vi "S2C_BldQuickView.vi"(8 "Error In":errorcluster) -> (0 "Error Out":errorcluster)   [LabVIEW 2015]
doc: "Detects an error and calls the error case to process the error."
uses:
  Globals/S2C_Globals.vi
  Globals/S2C_GlobalMenus.vi
panel:
  in  "QV-Exit":bool
  out "Init":bool
  in  "Selection":enum16{"Command", "Step", "Both"}(ring)=enum."Both"
  out "Window":string
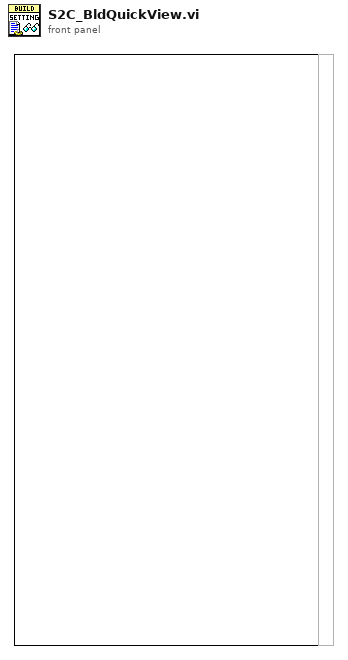
[diagram p1: front panel]
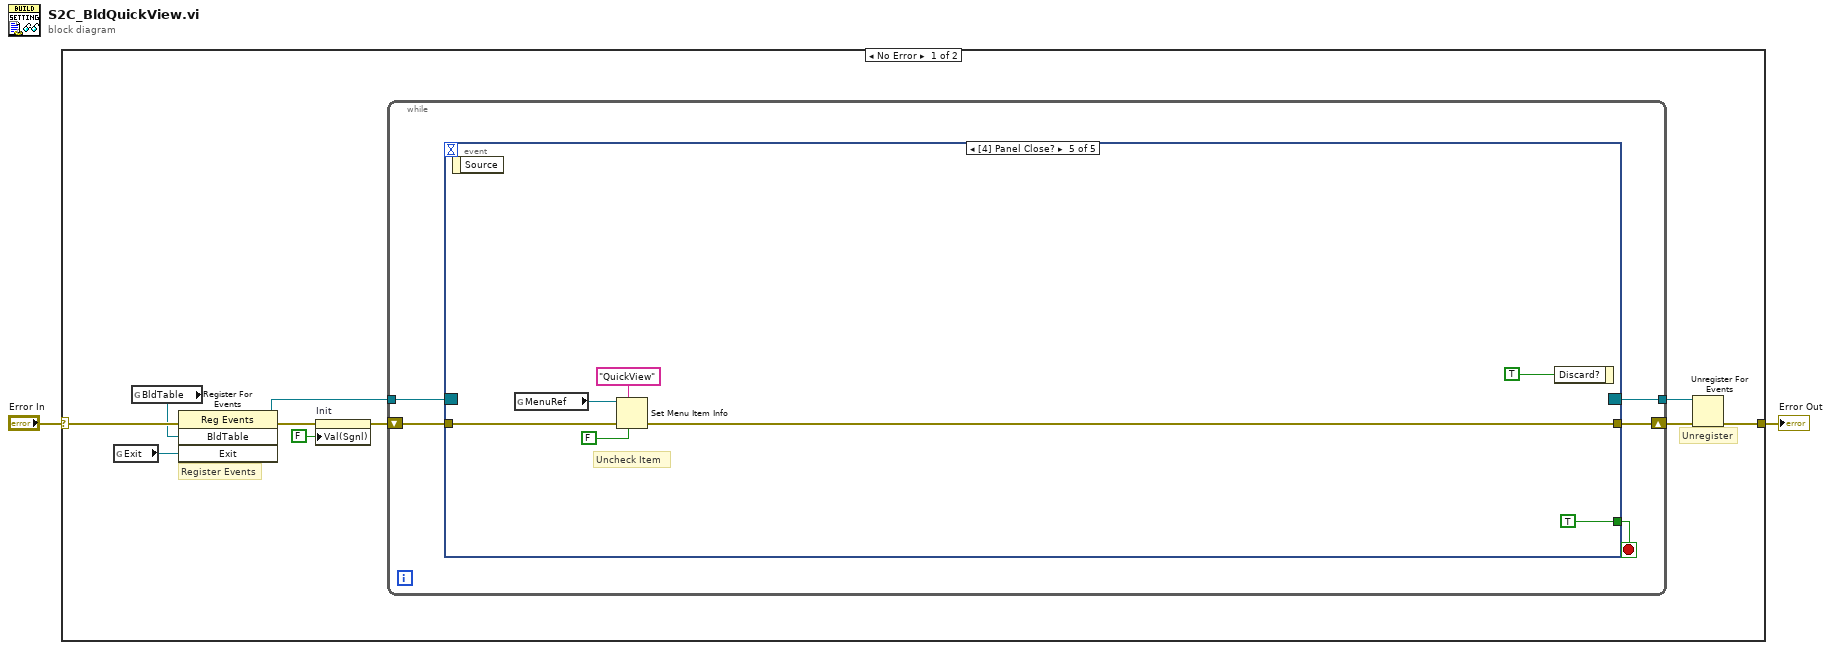
[diagram p0: block diagram]
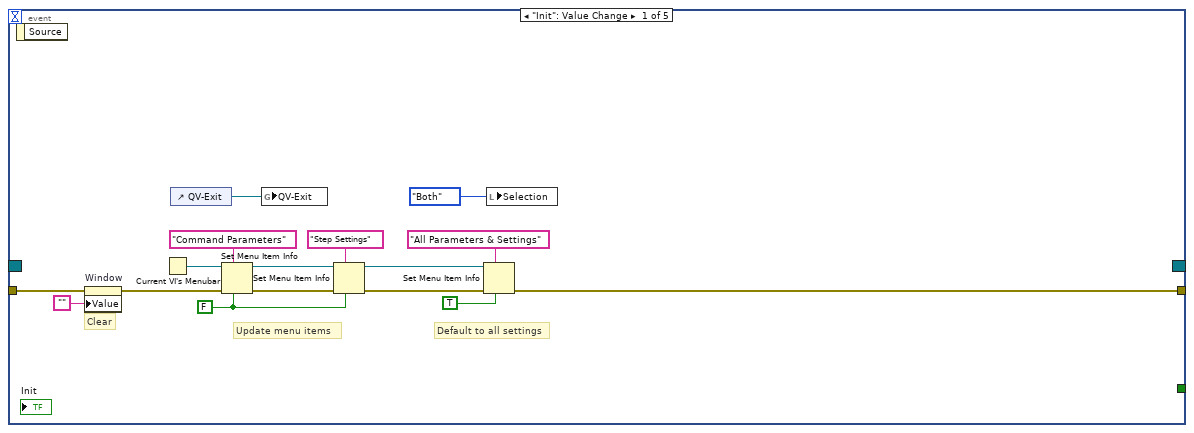
[diagram p2: hidden frame]
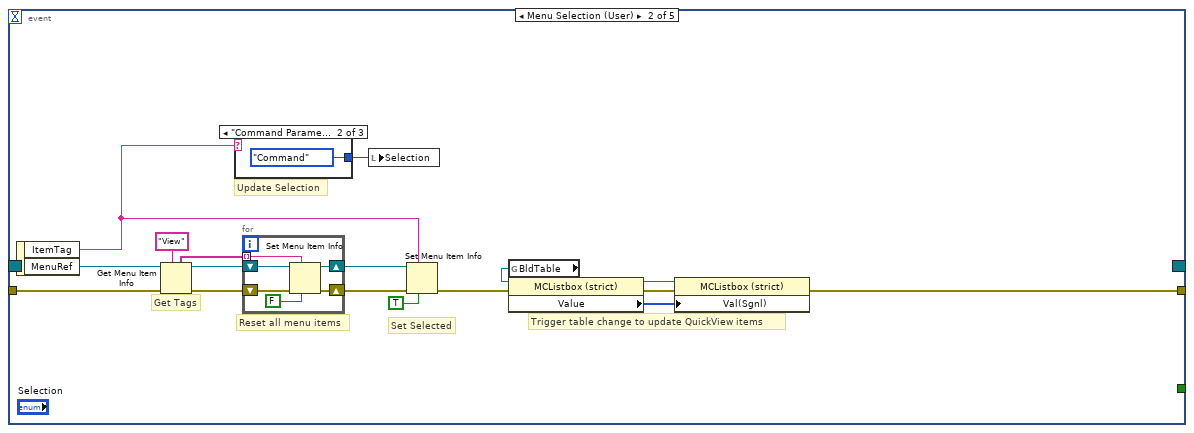
[diagram p3: hidden frame]
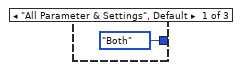
[diagram p4: hidden frame]
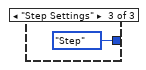
[diagram p5: hidden frame]
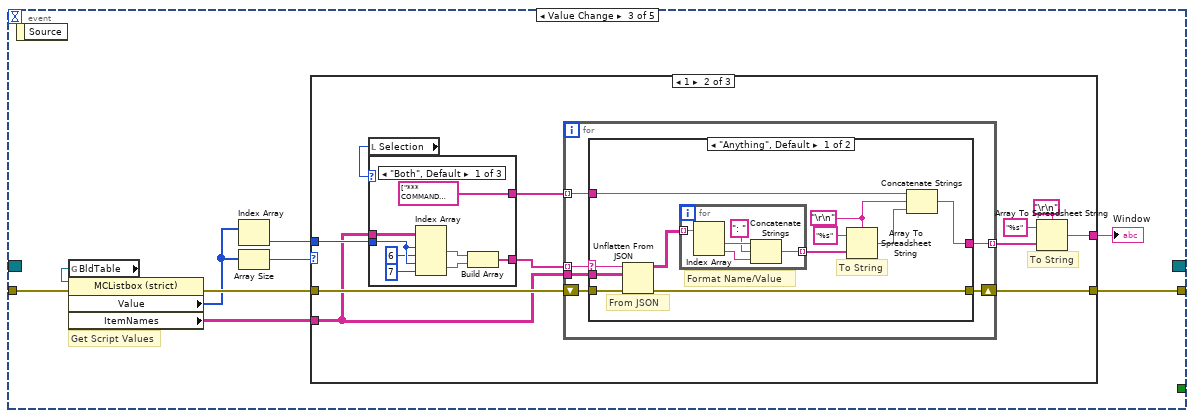
[diagram p6: hidden frame]
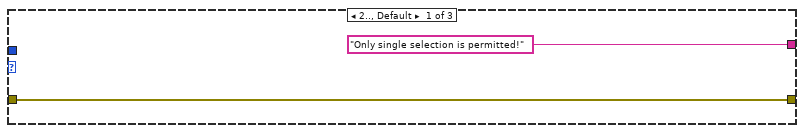
[diagram p7: hidden frame]
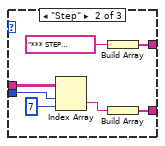
[diagram p8: hidden frame]
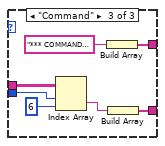
[diagram p9: hidden frame]
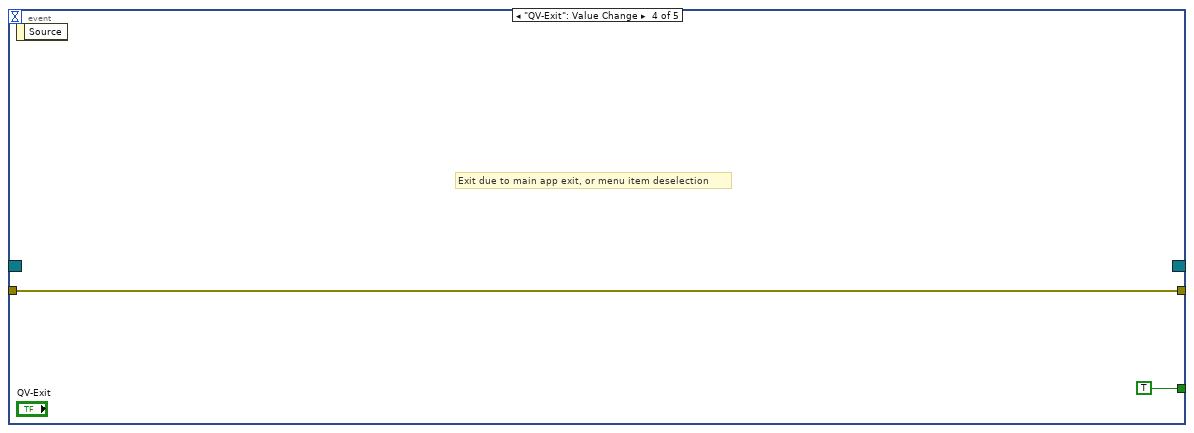
[diagram p12: hidden frame]
diagram:
  n1 = case shown="No Error" "Error In" {
    selector: "Error In" -> [w12 w136]
    tunnel: [w8 w136] -> w1
    frame No Error {
      # "Register Events"
      # "Unregister"
      n2 = global read "S2C_Globals.vi" "Exit"() -> (w3:refnum<vi>)
      n3 = global read "S2C_Globals.vi" "BldTable"() -> (w11:refnum<vi>)
      n4 = register-events(error in=w12, w11, w3) -> (reference out=w10:refnum<event-registration>, error out=w6:errorcluster)  [unwired: 1 in]
      n5 = property on="Init" class="Bool (strict)"(error in=w6, "Val(Sgnl)"=FALSE ("Value (Signaling)")) -> (error out=w4:errorcluster)  [unwired: 1 in, 1 out]
      n6 = while {
        shift-right: [w16] -> w9
        shift-left: w4 -> [w17]
        tunnel: w10 -> [w15]
        tunnel: [w14] -> w7
        stop <- w13 stop-if-true
        n7 = event shown="[4] Panel Close?" {
          selector: w15 -> [_ _ _ _ _]
          dyn-events: [_ _ _ _ _] -> w14
          timeout: _ -> [_ _ _ _ _]
          tunnel: w17 -> [w33 w50 w63 w129 w135]
          tunnel: [w20 w39 w68 w129 w135] -> w16
          tunnel: [_ _ _ TRUE TRUE] -> w13
          event "Init": Value Change {
            w22 = FALSE ("checked")
            # "Clear"
            # "Default to all settings"
            # "Update menu items"
            n8 = event-data() -> ()  [unwired: 1 in, 1 out]
            n9 = property on="Window" class="Str"(error in=w33, "Value"="") -> (error out=w31:errorcluster)  [unwired: 1 in, 1 out]
            n10 = Current VI's Menubar() -> (w30:refnum<k9>)
            n11 = control-ref of="QV-Exit"() -> (w18:refnum<vi>)
            n12 = Set Menu Item Info(6:w22, 7:"Command Parameters" ("item tag"), 8:w31, 11:w30) -> (0:w27:errorcluster, 3:w26:refnum<k9>)  [unwired: 3 in]
            n13 = global write "S2C_Globals.vi" "QV-Exit"(w18) -> ()
            n14 = Set Menu Item Info(6:w22, 7:"Step Settings" ("item tag"), 8:w27, 11:w26) -> (0:w24:errorcluster, 3:w23:refnum<k9>)  [unwired: 3 in]
            n15 = Set Menu Item Info(6:TRUE ("checked"), 7:"All Parameters & Settings" ("item tag"), 8:w24, 11:w23) -> (0:w20:errorcluster)  [unwired: 3 in, 1 out]
            n16 = local write "Selection"(enum16{"Command", "Step", "Both"}."Both" ("Selection")) -> ()
          }
          event Menu Selection (User) {
            # "Trigger table change to update QuickView items"
            # "Update Selection"
            # "Get Tags"
            # "Set Selected"
            # "Reset all menu items"
            n17 = event-data() -> ("ItemTag"=w41:string, "MenuRef"=w48:refnum<k9>)  [unwired: 1 in]
            n18 = Get Menu Item Info(7:"View" ("item tag"), 8:w50, 11:w48) -> (0:w49:errorcluster, 3:w47:refnum<k9>, 5:w44:string[])  [unwired: 4 out]
            n19 = case shown="\"Command Parameters\"" w41 {
              tunnel: [enum16{"Command", "Step", "Both"}."Both" ("Selection") enum16{"Command", "Step", "Both"}."Command" ("Selection") enum16{"Command", "Step", "Both"}."Step" ("Selection")] -> w46
              frame "All Parameter & Settings", Default {
              }
              frame "Command Parameters" {
              }
              frame "Step Settings" {
              }
            }
            n20 = for {
              shift-right: [w54] -> w43
              shift-left: w49 -> [w56]
              tunnel: w44 -> [w53] mode=indexing
              shift-right: [w51] -> w42
              shift-left: w47 -> [w55]
              n21 = Set Menu Item Info(6:FALSE ("checked"), 7:w53, 8:w56, 11:w55) -> (0:w54:errorcluster, 3:w51:refnum<k9>)  [unwired: 3 in]
            }
            n22 = local write "Selection"(w46) -> ()
            n23 = Set Menu Item Info(6:TRUE ("checked"), 7:w41, 8:w43, 11:w42) -> (0:w37:errorcluster)  [unwired: 3 in, 1 out]
            n24 = global read "S2C_Globals.vi" "BldTable"() -> (w38:refnum<vi>)
            n25 = property class="MCListbox (strict)"(reference=w38, error in=w37) -> (reference out=w35:refnum<vi>, error out=w36:errorcluster, "Value"=w34:i32[])
            n26 = property class="MCListbox (strict)"(reference=w35, error in=w36, "Val(Sgnl)"=w34) -> (error out=w39:errorcluster)  [unwired: 1 out]
          }
          event Value Change {
            # "Get Script Values"
            n27 = event-data() -> ()  [unwired: 1 in, 1 out]
            n28 = global read "S2C_Globals.vi" "BldTable"() -> (w64:refnum<vi>)
            n29 = property class="MCListbox (strict)"(reference=w64, error in=w63) -> (error out=w62:errorcluster, "Value"=w61:i32[], "ItemNames"=w60:string[][])  [unwired: 1 out]
            n30 = Index Array(array=w61) -> (element=w66:i32)  [unwired: 1 in]
            n31 = Array Size(array=w61) -> (size(s)=w67:i32)
            n32 = case shown="1" w67 {
              tunnel: w62 -> [w70 w74 w127]
              tunnel: [w70 w80 w127] -> w68
              tunnel: w66 -> [_ w81 _]
              tunnel: ["Only single selection is permitted!" ("spreadsheet string") w75 _] -> w65
              tunnel: w60 -> [_ w73 _]
              frame 2.., Default {
              }
              frame 1 {
                # "To String"
                n33 = local read "Selection"() -> (w72:enum16{"Command", "Step", "Both"})
                n34 = case shown="\"Both\", Default" w72 {
                  tunnel: w81 -> [w89 w96 w103]
                  tunnel: [w84 w93 w100] -> w79
                  tunnel: w73 -> [w83 w92 w99]
                  tunnel: [string[] ["*** COMMAND PARAMETERS ***", "*** STEP SETTINGS ***"] w90 w97] -> w71
                  frame "Both", Default {
                    n35 = Index Array(array=w83, index (row) #1=w89, index (col) #1=6 ("disabled index (col)"), index (row) #2=w89, index (col) #2=7 ("disabled index (col)")) -> (element #1=w86:string, element #2=w85:string)
                    n36 = Build Array(w86, w85) -> (w84:string[])
                  }
                  frame "Step" {
                    n37 = Index Array(array=w92, index (row)=w96, index (col)=7 ("disabled index (col)")) -> (element=w94:string)
                    n38 = Build Array("*** STEP SETTINGS ***") -> (w90:string[])
                    n39 = Build Array(w94) -> (w93:string[])
                  }
                  frame "Command" {
                    n40 = Index Array(array=w99, index (row)=w103, index (col)=6 ("disabled index (col)")) -> (element=w101:string)
                    n41 = Build Array("*** COMMAND PARAMETERS ***") -> (w97:string[])
                    n42 = Build Array(w101) -> (w100:string[])
                  }
                }
                n43 = for {
                  tunnel: w79 -> [w108] mode=indexing
                  tunnel: w73 -> [w106]
                  shift-right: [w107] -> w80
                  shift-left: w74 -> [w109]
                  tunnel: [w105] -> w78 mode=indexing
                  tunnel: w71 -> [w104] mode=indexing
                  n44 = case shown="\"Anything\", Default" w108 {
                    selector: w108 -> [w116 _]
                    tunnel: w109 -> [w118 w126]
                    tunnel: [w117 w126] -> w107
                    tunnel: w106 -> [w115 _]
                    tunnel: [w110 _] -> w105
                    tunnel: w104 -> [w113 _]
                    frame "Anything", Default {
                      w112 = "\r\n"
                      # "To String"
                      # "Format Name/Value"
                      # "From JSON"
                      n45 = Unflatten From JSON(JSON string=w116, type and defaults=w115, error in (no error)=w118) -> (value=w114:string[][], error out=w117:errorcluster)  [unwired: 4 in]
                      n46 = for {
                        tunnel: w114 -> [w121] mode=indexing
                        tunnel: [w124] -> w119 mode=indexing
                        n47 = Index Array(array=w121) -> (element #1=w123:string, element #2=w125:string)  [unwired: 2 in]
                        n48 = Concatenate Strings(w123, ": ", w125) -> (w124:string)
                      }
                      n49 = Array To Spreadsheet String(delimiter (Tab)=w112, array=w119, 3:"%s" ("format string")) -> (spreadsheet string=w111:string)
                      n50 = Concatenate Strings(w113, w112, w111) -> (w110:string)
                    }
                    frame "", "0" {
                      # "No settings available"
                    }
                  }
                }
                n51 = Array To Spreadsheet String(delimiter (Tab)="\r\n", array=w78, 3:"%s" ("format string")) -> (spreadsheet string=w75:string)
              }
              frame 0 {
              }
            }
            "Window" <- w65
          }
          event "QV-Exit": Value Change {
            # "Exit due to main app exit, or menu item deselection"
            n52 = event-data() -> ()  [unwired: 1 in, 1 out]
          }
          event Panel Close? {
            # "Uncheck Item"
            n53 = event-data() -> ()  [unwired: 1 in, 1 out]
            n54 = global read "S2C_GlobalMenus.vi" "MenuRef"() -> (w131:refnum<k9>)
            n55 = Set Menu Item Info(6:FALSE ("checked"), 7:"QuickView" ("item tag"), 11:w131) -> ()  [unwired: 4 in, 2 out]
            n56 = event-data("Discard?"=TRUE) -> ()  [unwired: 1 in, 1 out]
          }
        }
      }
      n57 = Unregister For Events(event registration refnum=w7, error in=w9) -> (error out=w8:errorcluster)
    }
    frame Error {
    }
  }
  "Error Out" <- w1
